vi "Get 1D Array Double.vi"(5 "use temporary file? (F)":bool, 7 "data type of variable":dbl[](array[numeric]), 8 "error in":errorcluster, 10 "variable name":string, 11 "GOLPI ref. in":T1={"pipe handle"={"lv_proc.dll file path"=path "", "process instance handle"=[], "debug mode"=FALSE, "debug data"=[]}, "fast read timeout [ms]"=500, "fast read settle time [ms]"=10, "fast read to multiple [ms]"=1, "max elements per input line"=100, "slow read timeout [ms]"=5000, "stdin double format specifier"="%_16e", "max elements per stdout output column"=100, "console mode bitstream"=FALSE, "bitstream first read timeout [ms]"=1000, "bitstream read timeout [ms]"=50, "struct transfer possible"=FALSE, "matlab mode"=FALSE, "var pipe write timeout [ms]"=5000, "variable pipe mode"=FALSE, "variable pipe buffer size [Bytes]"=10000000, "variable pipe block size [Bytes]"=1000000} {"variable pipe block size [Bytes]" format="%.0p"; "variable pipe buffer size [Bytes]" format="%.0p"}) -> (0 "error out":errorcluster, 2 "value":dbl[](array[numeric]) format="%.2f", 3 "GOLPI ref. out":T1={"pipe handle"={"lv_proc.dll file path"=path "", "process instance handle"=[], "debug mode"=FALSE, "debug data"=[]}, "fast read timeout [ms]"=500, "fast read settle time [ms]"=10, "fast read to multiple [ms]"=1, "max elements per input line"=100, "slow read timeout [ms]"=5000, "stdin double format specifier"="%_16e", "max elements per stdout output column"=100, "console mode bitstream"=FALSE, "bitstream first read timeout [ms]"=1000, "bitstream read timeout [ms]"=50, "struct transfer possible"=FALSE, "matlab mode"=FALSE, "var pipe write timeout [ms]"=5000, "variable pipe mode"=FALSE, "variable pipe buffer size [Bytes]"=10000000, "variable pipe block size [Bytes]"=1000000} {"variable pipe block size [Bytes]" format="%.0p"; "variable pipe buffer size [Bytes]" format="%.0p"})   [LabVIEW 2020, in "GOLPI library.lvlib"]
doc: "Part of polymorph Get Variable.vi"
uses:
  GOLPI library.lvlib
  Public/GOLPI reference Type Def.ctl
  LV Process source distribution/Pipe Handle.ctl
  Type Definitions/Custom Error Codes Enum Type Def.vi
  Type Definitions/Bitstream Data Type.ctl
  LV Process source distribution/LV Process library.lvlib
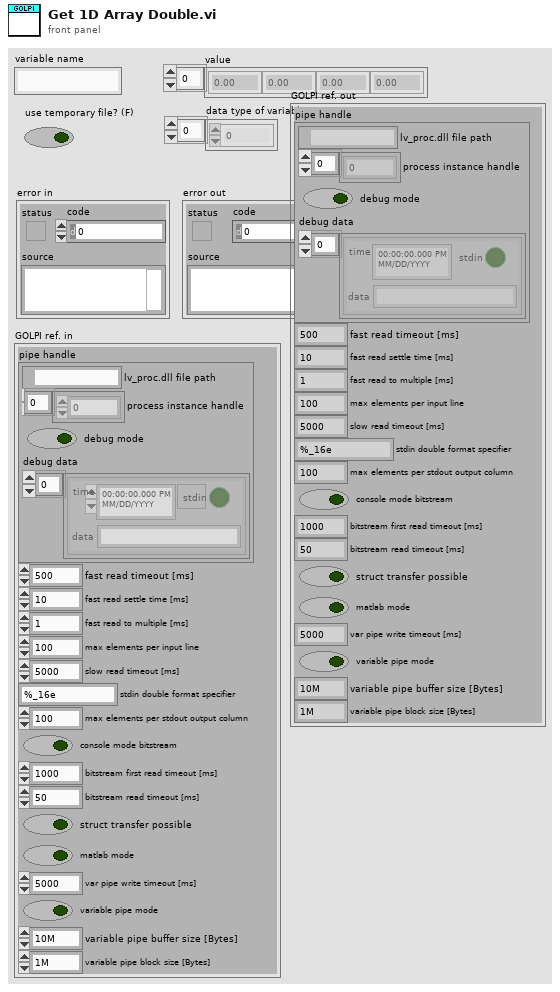
[diagram p1: front panel]
types:
  T1 = typedef "GOLPI library.lvlib/GOLPI reference Type Def.ctl" = cluster{"pipe handle":T2, "fast read timeout [ms]":u32, "fast read settle time [ms]":u32, "fast read to multiple [ms]":u32, "max elements per input line":u32, "slow read timeout [ms]":u32, "stdin double format specifier":string, "max elements per stdout output column":u32, "console mode bitstream":bool, "bitstream first read timeout [ms]":u32, "bitstream read timeout [ms]":u32, "struct transfer possible":bool, "matlab mode":bool, "var pipe write timeout [ms]":u32, "variable pipe mode":bool, "variable pipe buffer size [Bytes]":u32, "variable pipe block size [Bytes]":u32}
  T2 = typedef "LV Process library.lvlib/Pipe Handle.ctl" = cluster{"lv_proc.dll file path":path, "process instance handle":u32[], "debug mode":bool, "debug data":cluster{"time":timestamp, "stdin":bool, "data":string}[]}
  T3 = typedef "GOLPI library.lvlib/Custom Error Codes Enum Type Def.vi" = enum16{"no error", "00 working directory PAR1 missing", "01 octave binary PAR1 missing", "02 octave report error PAR1", "03 empty output last cmd PAR1", "04 missing temporary file PAR1", "05 pwd PAR 1 not exist", "06 oct package not installed", "07 octave default binary missing", "10 var PAR1 not string, vect", "11 var PAR1 not num, scal, ~compl", "12 var PAR1 not num, scal, compl", "13 var PAR1 not num, vect, ~compl", "14 var PAR1 not num, vect, compl", "15 var PAR1 not num, mat, ~compl", "16 var PAR1 not num, mat, ~compl", "30 read timeout", "60 bitstream transport failed", "61 bitstream decode error PAR1", "62 bitstream cannot be set", "70 struct transfer not possible", "80 struct: cluster elem. PAR1 not implem.", "81 struct: structure field PAR1 not implem.", "82 struct: size mismatch of PAR1", "83 struct: type mismatch of PAR1", "98 internal error", "99 not finished", "90 Not supported in Matlab mode", "91 Matlab variable transfer error", "92 Matlab Script Error", "100 Variable Pipe Mode cannot be set"}
  T4 = typedef "GOLPI library.lvlib/Bitstream Data Type.ctl" = enum16{"dummy", "int", "uint", "float", "complex", "str", "real numeric"}
  T5 = typedef "GOLPI library.lvlib/Transfer Mode.ctl" = enum16{"Matlab", "stdio", "temp file", "bitstream", "pipe"}
  T6 = typedef "GOLPI library.lvlib/Bitstream Data.ctl" = cluster{"double":dbl[][], "cplx double":cdb[][], "int64":i64[][], "uint64":u64[][], "str":string[], "data type":T4}
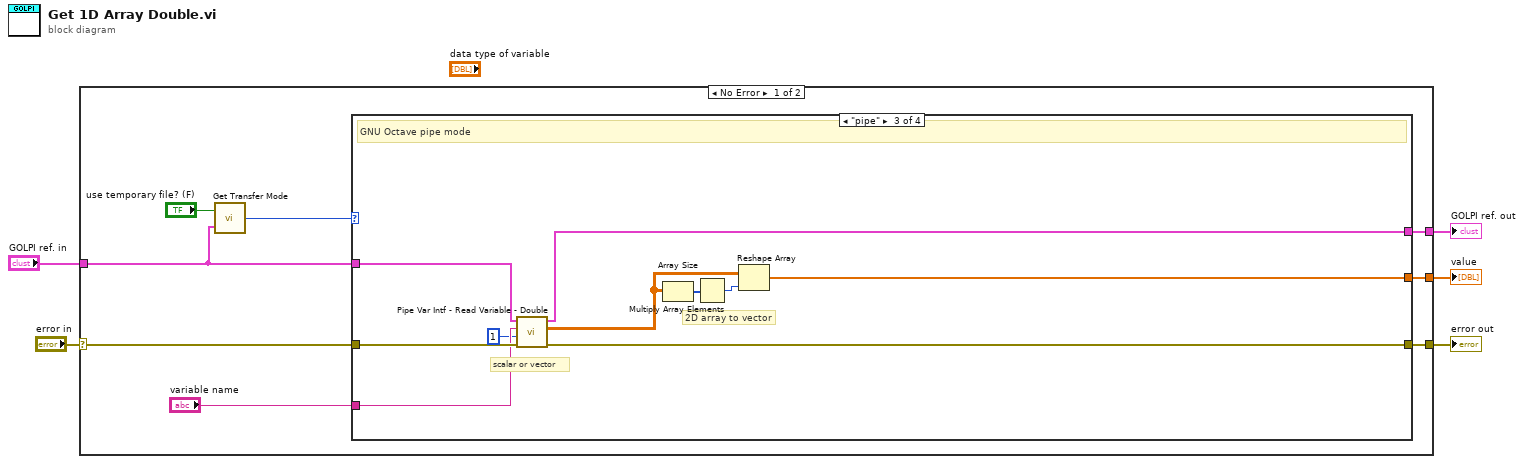
[diagram p0: block diagram]
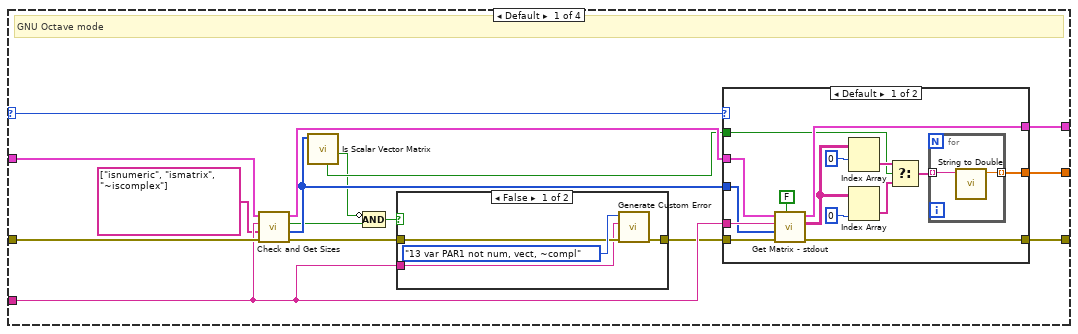
[diagram p2: hidden frame]
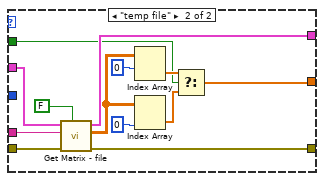
[diagram p3: hidden frame]
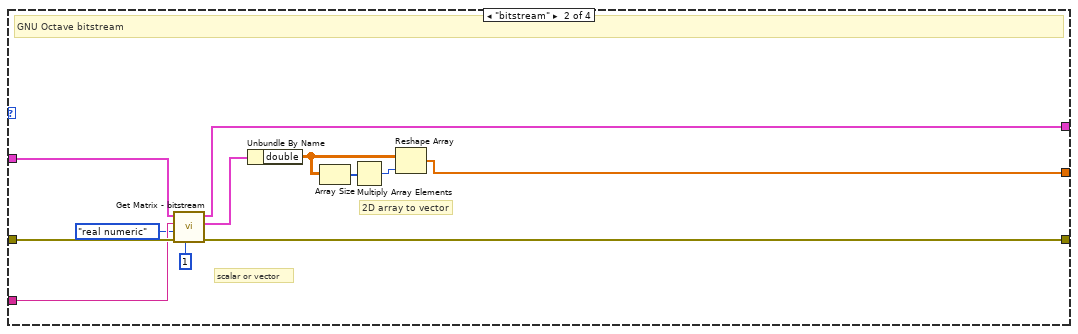
[diagram p5: hidden frame]
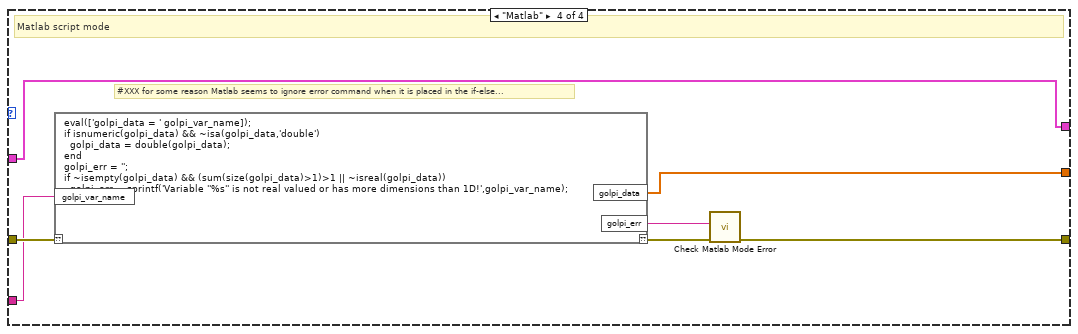
[diagram p6: hidden frame]
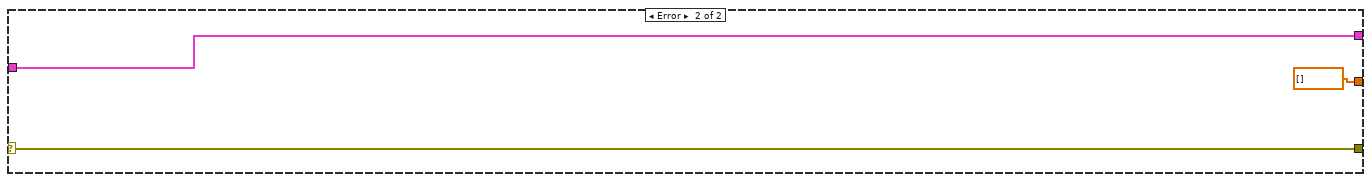
[diagram p7: hidden frame]
diagram:
  n1 = case shown="No Error" "error in" {
    selector: "error in" -> [w12 w96]
    tunnel: [w11 w96] -> w5
    tunnel: [w13 dbl[] [] ("value")] -> w3
    tunnel: "GOLPI ref. in" -> [w7 w94]
    tunnel: [w9 w94] -> w1
    frame No Error {
      n2 = call "Get Transfer Mode.vi"("GOLPI ref."=w7, "use temporary file? (F)"="use temporary file? (F)") -> ("mode"=w6:T5)
      n3 = case shown="\"pipe\"" w6 {
        selector: w6 -> [w14 _ _ _]
        tunnel: [w29 w76 w86 w90] -> w13
        tunnel: w12 -> [w28 w75 w85 w93]
        tunnel: [w27 w74 w84 w88] -> w11
        tunnel: "variable name" -> [w26 w73 w83 w91]
        tunnel: [w25 w72 w82 w92] -> w9
        tunnel: w7 -> [w24 w71 w81 w92]
        frame Default {
          # "GNU Octave mode"
          n4 = call "Check and Get Sizes.vi"("error in (no error)"=w28, "test commands"=string[] ["isnumeric", "ismatrix", "~iscomplex"], "variable name"=w26, "GOLPI ref. in"=w24) -> ("error out"=w23:errorcluster, "octave sizes"=w19:i32[], "all tests OK?"=w16:bool, "GOLPI ref. out"=w21:T1)  [unwired: 4 in]
          n5 = call "Is Scalar Vector Matrix.vi"("octave sizes"=w19) -> ("is matrix?"=w15:bool, "row vector?"=w18:bool)  [unwired: 5 in, 4 out]
          n6 = Compound Arithmetic op=AND(invert w15, w16) -> (w17:bool)
          n7 = case shown="False" w17 {
            tunnel: w23 -> [w62 w64]
            tunnel: [w61 w64] -> w20
            tunnel: w26 -> [w60 _]
            frame False {
              n8 = call "Generate Custom Error.vi"("error in"=w62, "PAR1"=w60, "GOLPI error"=Custom_Error_Codes_Enum_Type_Def.vi."13 var PAR1 not num, vect, ~compl" ("Enum")) -> ("error out"=w61:errorcluster)  [unwired: 8 in]
            }
            frame True {
            }
          }
          n9 = case shown="Default" w14 {
            tunnel: [w30 w52] -> w29
            tunnel: w21 -> [w37 w58]
            tunnel: [w33 w57] -> w25
            tunnel: w20 -> [w38 w55]
            tunnel: [w34 w54] -> w27
            tunnel: w26 -> [w36 w56]
            tunnel: w19 -> [w35 _]
            tunnel: w18 -> [w32 w47]
            frame Default {
              n10 = call "Get Matrix - stdout.vi"("is string?"=FALSE ("is string"), "error in (no error)"=w38, "octave sizes"=w35, "variable name"=w36, "GOLPI ref. in"=w37) -> ("error out"=w34:errorcluster, "array"=w39:string[][], "GOLPI ref. out"=w33:T1)  [unwired: 4 in]
              n11 = Index Array(array=w39, index (row)=0) -> (element=w41:string[])  [unwired: 1 in]
              n12 = Index Array(array=w39, index (col)=0 ("disabled index (col)")) -> (element=w40:string[])  [unwired: 1 in]
              n13 = Select(t=w41, s=w32, f=w40) -> (s? t:f=w31:string[])
              n14 = for {
                tunnel: w31 -> [w46] mode=indexing
                tunnel: [w45] -> w30 mode=indexing
                n15 = call "String to Double.vi"("string"=w46) -> ("number"=w45:dbl)  [unwired: 10 in]
              }
            }
            frame "temp file" {
              n16 = call "Get Matrix - file.vi"("is string?"=FALSE ("is string"), "error in (no error)"=w55, "variable name"=w56, "GOLPI ref. in"=w58) -> ("error out"=w54:errorcluster, "double array"=w50:dbl[][], "GOLPI ref. out"=w57:T1)  [unwired: 3 in, 2 out]
              n17 = Index Array(array=w50, index (row)=0) -> (element=w51:dbl[])  [unwired: 1 in]
              n18 = Index Array(array=w50, index (col)=0 ("disabled index (col)")) -> (element=w53:dbl[])  [unwired: 1 in]
              n19 = Select(t=w51, s=w47, f=w53) -> (s? t:f=w52:dbl[])
            }
          }
        }
        frame "bitstream" {
          # "2D array to vector"
          # "scalar or vector"
          # "GNU Octave bitstream"
          n20 = call "Get Matrix - bitstream.vi"("max dimensions (0: scalar)"=1, "error in (no error)"=w75, "data type"=Bitstream_Data_Type."real numeric", "variable name"=w73, "GOLPI ref. in"=w71) -> ("error out"=w74:errorcluster, "data"=w68:T6, "GOLPI ref. out"=w72:T1)  [unwired: 4 in]
          n21 = Unbundle By Name(w68) -> ("double"=w67:dbl[][])
          n22 = Array Size(array=w67) -> (size(s)=w66:i32[])
          n23 = Multiply Array Elements(1:w66) -> (0:w65:i32)
          n24 = Reshape Array(w67, w65) -> (w76:dbl[])
        }
        frame "pipe" {
          # "2D array to vector"
          # "scalar or vector"
          # "GNU Octave pipe mode"
          n25 = call "Pipe Var Intf - Read Variable - Double.vi"("error in (no error)"=w85, "max dims (0: scalar)"=1 ("max dimensions (0: scalar)"), "variable name"=w83, "GOLPI ref. in"=w81) -> ("error out"=w84:errorcluster, "data out"=w77:dbl[][], "GOLPI ref. out"=w82:T1)  [unwired: 5 in]
          n26 = Array Size(array=w77) -> (size(s)=w79:i32[])
          n27 = Multiply Array Elements(1:w79) -> (0:w78:i32)
          n28 = Reshape Array(w77, w78) -> (w86:dbl[])
        }
        frame "Matlab" {
          # "#XXX for some reason Matlab seems to ignore error command when it is placed in the if-else..."
          # "Matlab script mode"
          n29 = script code="eval(['golpi_data = ' golpi_var_name]);\nif isnumeric(golpi_data) && ~isa(golpi_data,'double')\n  golpi_data = double(golpi_data);\nend\ngolpi_err = '';\nif ~isempty(golpi_data) && (sum(size(golpi_data)>1)>1 || ~isreal(golpi_data))\n  golpi_err = sprintf('Variable ''%s'' is not real valued or has more dimensions than 1D!',golpi_var_name);\nend"("??"=w93, "golpi_var_name"=w91) -> ("??"=w89:errorcluster, "golpi_data"=w90:dbl[], "golpi_err"=w87:string)
          n30 = call "Check Matlab Mode Error.vi"("error in"=w89, "custom error string (empty)"=w87) -> ("error out"=w88:errorcluster)  [unwired: 9 in]
        }
      }
    }
    frame Error {
    }
  }
  "value" <- w3
  "error out" <- w5
  "GOLPI ref. out" <- w1
